vi "Laser_toggles_SAE.vi"() -> ()   [LabVIEW 2020]
uses:
  type_defs/Laser_toggles_typedef.ctl
panel:
  in  "stop":bool
  out "Laser Toggles OUT":T1 {"Laser 488 order selection" items=["Not active", "1", "2", "3", "4"]; "Laser 642 order selection" items=["Not active", "1", "2", "3", "4"]; "Laser 595 order selection" items=["Not active", "1", "2", "3", "4"]; "Laser 560 order selection" items=["Not active", "1", "2", "3", "4"]; "Laser 642 nm power" min=0.0 max=5.0 scale=0.0..100.0; "Laser 595 nm power" min=0.0 max=5.0 scale=0.0..100.0; "Laser 560 nm power" min=0.0 max=5.0 scale=0.0..100.0; "Laser 488 nm power" min=0.0 max=5.0 scale=0.0..100.0}
  in  "Laser Toggles IN":T1 {"Laser 488 order selection" items=["Not active", "1", "2", "3", "4"]; "Laser 642 order selection" items=["Not active", "1", "2", "3", "4"]; "Laser 595 order selection" items=["Not active", "1", "2", "3", "4"]; "Laser 560 order selection" items=["Not active", "1", "2", "3", "4"]; "Laser 642 nm power" min=0.0 max=5.0 scale=0.0..100.0; "Laser 595 nm power" min=0.0 max=5.0 scale=0.0..100.0; "Laser 560 nm power" min=0.0 max=5.0 scale=0.0..100.0; "Laser 488 nm power" min=0.0 max=5.0 scale=0.0..100.0}
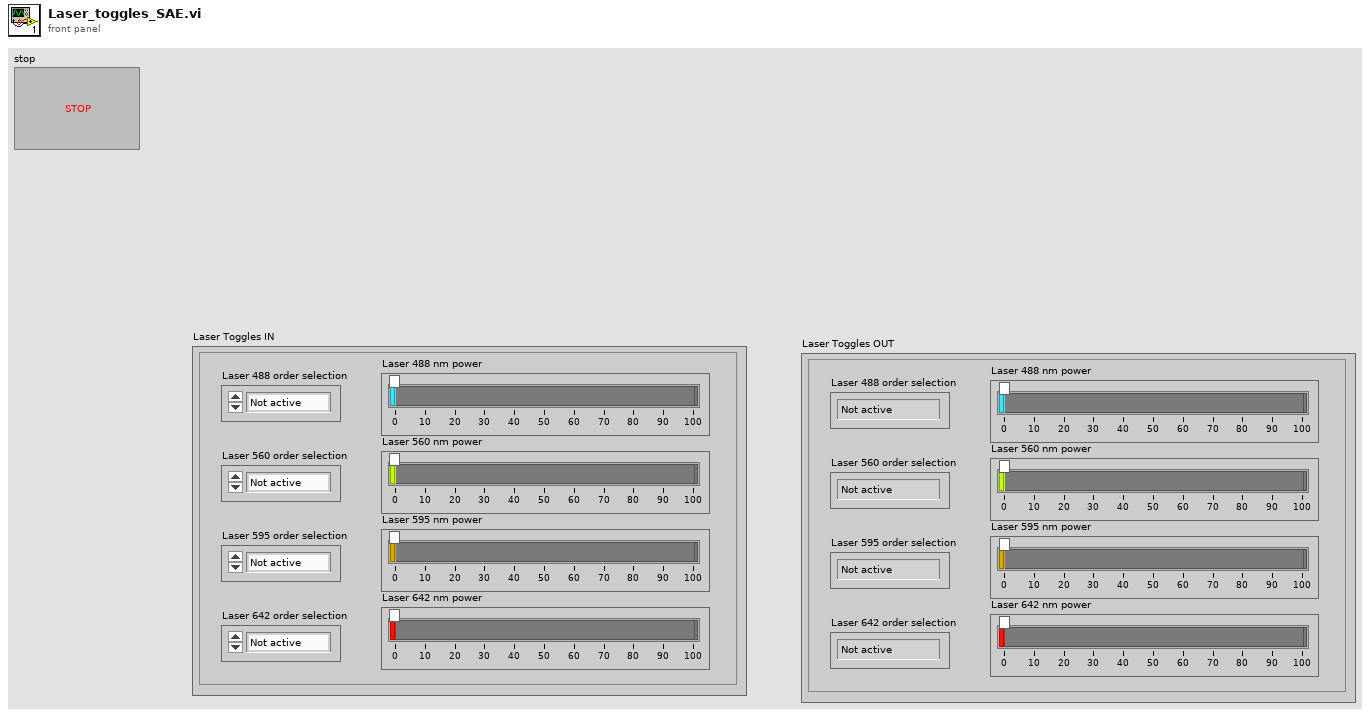
[diagram p1: front panel]
types:
  T1 = typedef "Laser_toggles_typedef.ctl" = cluster{"Laser 488 nm power":dbl, "Laser 560 nm power":dbl, "Laser 595 nm power":dbl, "Laser 642 nm power":dbl, "Laser 560 order selection":u16, "Laser 595 order selection":u16, "Laser 642 order selection":u16, "Laser 488 order selection":u16}
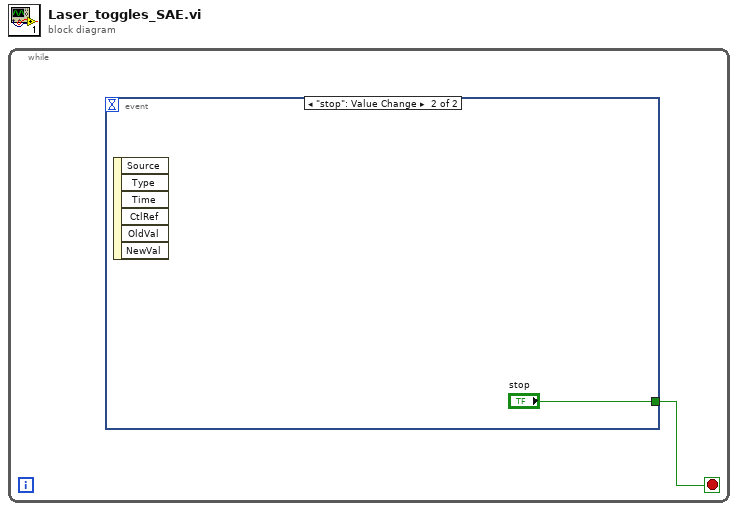
[diagram p0: block diagram]
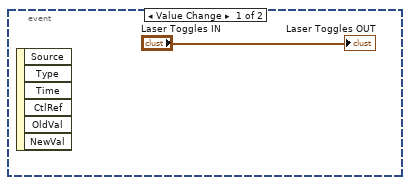
[diagram p2: hidden frame]
diagram:
  n1 = while {
    stop <- w1 stop-if-true
    n2 = event shown="[1] \"stop\": Value Change" {
      selector: _ -> [_ _]
      dyn-events: _ -> [_ _]
      timeout: _ -> [_ _]
      tunnel: [_ "stop"] -> w1
      event Value Change {
        n3 = event-data() -> ()  [unwired: 1 in, 6 out]
        "Laser Toggles OUT" <- "Laser Toggles IN"
      }
      event "stop": Value Change {
        n4 = event-data() -> ()  [unwired: 1 in, 6 out]
      }
    }
  }
